vi "Find Setting String.vi"(9 "String In":string, 11 "Delimiter In":string) -> (1 "Greater than 1 Out":bool, 2 "Array Count Out":i32, 3 "String Array Out":string[](array[string]))   [LabVIEW 2026]
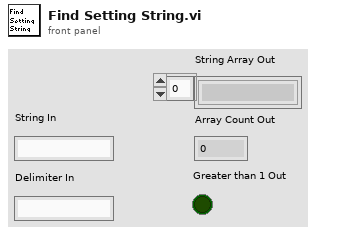
[diagram p1: front panel]
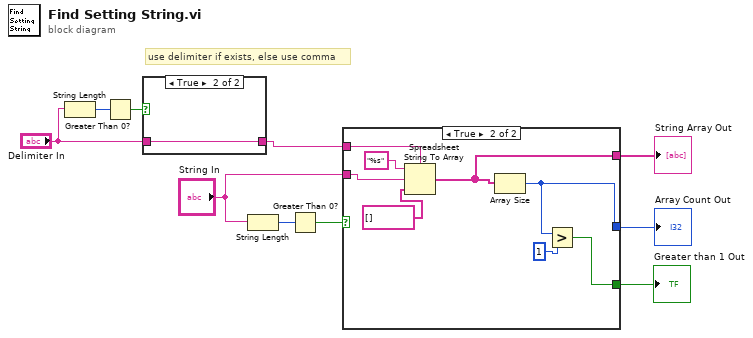
[diagram p0: block diagram]
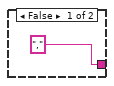
[diagram p2: hidden frame]
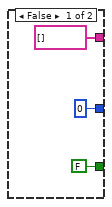
[diagram p3: hidden frame]
diagram:
  # "use delimiter if exists, else use comma"
  n1 = String Length(string="Delimiter In") -> (length=w2:i32)
  n2 = Greater Than 0?(x=w2) -> (x > 0?=w3:bool)
  n3 = case shown="True" w3 {
    tunnel: "Delimiter In" -> [_ w12]
    tunnel: ["," w12] -> w1
    frame False {
    }
    frame True {
    }
  }
  n4 = String Length(string="String In") -> (length=w9:i32)
  n5 = Greater Than 0?(x=w9) -> (x > 0?=w8:bool)
  n6 = case shown="True" w8 {
    tunnel: "String In" -> [_ w22]
    tunnel: w1 -> [_ w23]
    tunnel: [0 w19] -> w7
    tunnel: [FALSE w17] -> w6
    tunnel: [string[] [] w16] -> w5
    frame False {
    }
    frame True {
      n7 = Spreadsheet String To Array(delimiter (Tab)=w23, format string="%s", spreadsheet string=w22, array type (2D Dbl)=string[] []) -> (array=w16:string[])
      n8 = Array Size(array=w16) -> (size(s)=w19:i32)
      n9 = Greater?(x=w19, y=1) -> (0:w17:bool)
    }
  }
  "Array Count Out" <- w7
  "Greater than 1 Out" <- w6
  "String Array Out" <- w5
